vi "Error Calculations.vi"(1 "Eta_ref":dbl[](array[numeric])=[0.0, 0.0, 0.0, 0.0, 0.0, 0.0], 2 "Eta":dbl[](array[numeric])=[0.0, 0.0, 0.0, 0.0, 0.0, 0.0]) -> (0 "error":dbl[](array[numeric]))   [LabVIEW 2014]
uses:
  <vilib>/imath/engines/lvmath2/RunTimeEngine/IndexRead/NIMS V(S).vi
  <instcachedir>/0/NIMS V(S)_0488751826AF41519A22953C041130DC.lvgen/NIMS V(S)_0488751826AF41519A22953C041130DC_000.vi
  <vilib>/imath/engines/lvmath2/RunTimeEngine/ErrorHandling/NIMS_Create Error From Enums.vi
  <vilib>/imathl/engines/lvmath/Functions/Error Handling/Create Error.vi
  <vilib>/imath/engines/lvmath2/RunTimeEngine/IndexReplace/NIMS V(S)=S.vi
  <instcachedir>/0/NIMS V(S)=S_2D52C4EC15D8415E870AEE69FB516CCA.lvgen/NIMS V(S)=S_2D52C4EC15D8415E870AEE69FB516CCA_000.vi
  <vilib>/imath/engines/lvmath2/RunTimeEngine/ArithmeticOperatorToken/NIMS_ArithmeticOperator_minus.vi
  <instcachedir>/0/NIMS_ArithmeticOperator_minus_39C0593E74DA4138ACA2AB742906488D.lvgen/NIMS_ArithmeticOperator_minus_39C0593E74DA4138ACA2AB742906488D_003.vi
  <vilib>/imath/engines/lvmath2/RunTimeEngine/NodeEndStatement/NIMS_NodeEndStatement_Output.vi
  <instcachedir>/0/NIMS_NodeEndStatement_Output_53EC0D466D134D7ABD903AC30B43404B.lvgen/NIMS_NodeEndStatement_Output_53EC0D466D134D7ABD903AC30B43404B_005.vi
  <vilib>/imath/engines/lvmath2/RunTimeEngine/ErrorHandling/NIMS_Finalize Error.vi
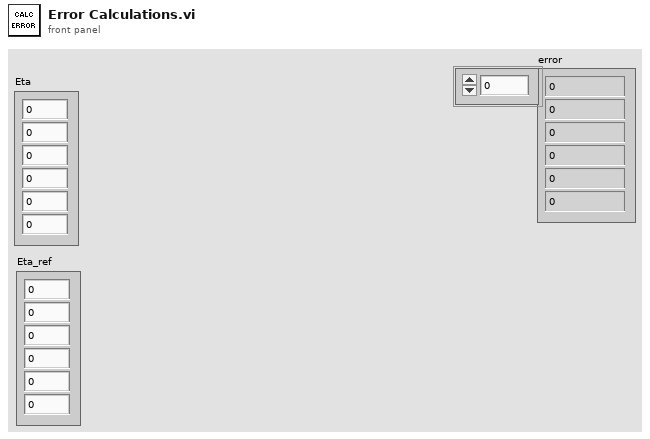
[diagram p1: front panel]
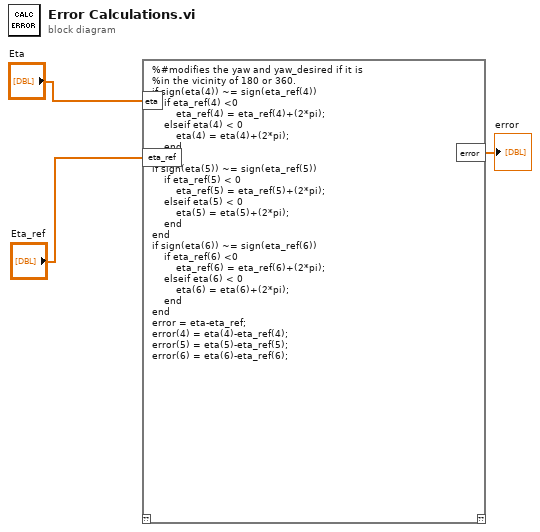
[diagram p0: block diagram]
diagram:
  n1 = mathscript code="%#modifies the yaw and yaw_desired if it is \n%in the vicinity of 180 or 360.\nif sign(eta(4)) ~= sign(eta_ref(4))\n    if eta_ref(4) <0\n        eta_ref(4) = eta_ref(4)+(2*pi);\n    elseif eta(4) < 0\n        eta(4) = eta(4)+(2*pi);\n    end    \nend\nif sign(eta(5)) ~= sign(eta_ref(5))\n    if eta_ref(5) < 0\n        eta_ref(5) = eta_ref(5)+(2*pi);\n    elseif eta(5) < 0\n        eta(5) = eta(5)+(2*pi);\n    end    \nend\nif sign(eta(6)) ~= sign(eta_ref(6))\n    if eta_ref(6) <0\n        eta_ref(6) = eta_ref(6)+(2*pi);\n    elseif eta(6) < 0\n        eta(6) = eta(6)+(2*pi);\n    end    \nend\nerror = eta-eta_ref;\nerror(4) = eta(4)-eta_ref(4);\nerror(5) = eta(5)-eta_ref(5);\nerror(6) = eta(6)-eta_ref(6);"("eta"="Eta", "eta_ref"="Eta_ref") -> ("error"=→"error":dbl[])  [unwired: 1 in, 1 out]
